vi "CreateEventGUI.vi"(8 "error in (no error)":errorcluster, 11 "DQMH_Modules":refnum<class "DQMHModuleNode.lvclass">[](array[class])) -> (0 "error out":errorcluster)   [LabVIEW 2016, in "DQMH_API.lvclass"]
uses:
  <resource>/Framework/Providers/Open_GDS/UML/DQMH_API_class/DQMH_API.lvclass
  <resource>/Framework/Providers/Open_GDS/UML/DQMHModuleNode_class/DQMHModuleNode.lvclass
  <resource>/Framework/Providers/Open_GDS/UML/DQMH_API_class/ModuleCreationType.ctl
  <resource>/Framework/Providers/Open_GDS/UML/DQMH_API_class/EventCreationType.ctl
  <resource>/Framework/Providers/Open_GDS/UML/DQMHModuleNode_class/EventType.ctl
  <vilib>/Utility/traverseref.llb/TRef TravTarget.ctl
panel:
  in  "Tree":string(tree) caption="Double click on event to create it"
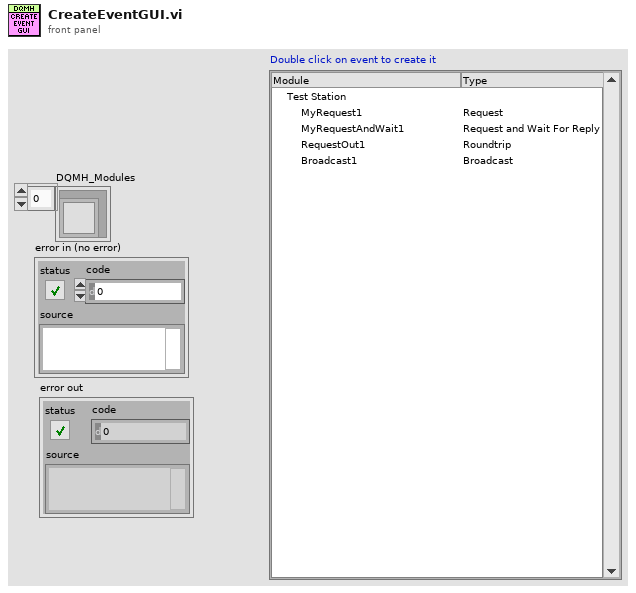
[diagram p1: front panel]
types:
  T1 = typedef "DQMH_API.lvclass/ModuleCreationType.ctl" = cluster{"LibraryName":string, "Events":T2[]}
  T2 = typedef "DQMH_API.lvclass/EventCreationType.ctl" = cluster{"Type":T3, "RequestName":string, "BroadcastName":string}
  T3 = typedef "DQMHModuleNode.lvclass/EventType.ctl" = enum16{"Request", "Request and Wait For Reply", "Roundtrip", "Broadcast"}
  T4 = cluster{"ModulesAndEvents":T1[], "EventExists":cluster{bool[]}[]}
  T5 = cluster{"Tag":string, "Cancelled":bool, "ModulesAndEvents":T1[], "ExistingEventPerModule":cluster{"Event Info":cluster{"Event VI Path":path, "Argument Path":path, "Wait Argument Path":path, "Event Arg Owner":i32, "Event Name":string, "Type":enum16{"Request", "Broadcast", "Both"}}[]}[], "EventExists":cluster{bool[]}[], "EventsCreated":cluster{bool[]}[], "DqmhCreateEventDialogRef":refnum<vi>, "Event":refnum<event-registration>, "WaitForCreation":bool, "ApplicationRef":refnum<vi>, "NewEventSubVI":refnum<vi>, "DQMH VIs":refnum<vi>[]}
  T6 = typedef "TRef TravTarget.ctl" = enum16{"FP", "BD", "Other"}
  T7 = cluster{"Event Info":cluster{"Event VI Path":path, "Argument Path":path, "Wait Argument Path":path, "Event Arg Owner":i32, "Event Name":string, "Type":enum16{"Request", "Broadcast", "Both"}}[]}[]
  T8 = cluster{"LibraryName":string, "Events":cluster{"Type":enum16{"Request", "Request and Wait For Reply", "Roundtrip", "Broadcast"}, "RequestName":string, "BroadcastName":string}[]}[]
  T9 = enum16{"Both", "Singleton Only", "Cloneable Only"}
  T10 = cluster{"Left Cell String":string, "Child Text":string[], "Child Tag":string, "Item Indent":i32, "Child Only?":bool, "Glyph Index":i32}
  T11 = enum32{"Bad", "Idle", "Run top level", "Running"}
  T12 = cluster{"Name":string, "Library":refnum<vi>, "Library Owning App":refnum<vi>, "Library Owning Folder":path, "Module Type":enum16{"Singleton", "Cloneable"}, "Public API Requests Folder":refnum<vi>, "Public API Requests Arguments Folder":refnum<vi>, "Broadcasts Folder":refnum<vi>, "Broadcasts Arguments Folder":refnum<vi>, "Obtain Broadcast Events VI":refnum<vi>, "Destroy Broadcast Events VI":refnum<vi>, "Obtain Request Events VI":refnum<vi>, "Destroy Request Events VI":refnum<vi>, "Request Events Cluster CTL":refnum<vi>, "Broadcast Events Cluster CTL":refnum<vi>, "Module Timeout VI":refnum<vi>, "Module Name VI":refnum<vi>, "Status Updated VI":refnum<vi>, "Module Not Running Error Constant VI":refnum<vi>}[]
  T13 = cluster{"Name":string, "Library":refnum<vi>, "Library Owning App":refnum<vi>, "Library Owning Folder":path, "Module Type":enum16{"Singleton", "Cloneable"}, "Public API Requests Folder":refnum<vi>, "Public API Requests Arguments Folder":refnum<vi>, "Broadcasts Folder":refnum<vi>, "Broadcasts Arguments Folder":refnum<vi>, "Obtain Broadcast Events VI":refnum<vi>, "Destroy Broadcast Events VI":refnum<vi>, "Obtain Request Events VI":refnum<vi>, "Destroy Request Events VI":refnum<vi>, "Request Events Cluster CTL":refnum<vi>, "Broadcast Events Cluster CTL":refnum<vi>, "Module Timeout VI":refnum<vi>, "Module Name VI":refnum<vi>, "Status Updated VI":refnum<vi>, "Module Not Running Error Constant VI":refnum<vi>}
  T14 = cluster{"Event VI Path":path, "Argument Path":path, "Wait Argument Path":path, "Event Arg Owner":i32, "Event Name":string, "Type":enum16{"Request", "Broadcast", "Both"}}[]
  T15 = cluster{"Event Info":cluster{"Event VI Path":path, "Argument Path":path, "Wait Argument Path":path, "Event Arg Owner":i32, "Event Name":string, "Type":enum16{"Request", "Broadcast", "Both"}}[]}
  T16 = typedef "LVRectTypeDef.ctl" = cluster{"Left":i16, "Top":i16, "Right":i16, "Bottom":i16}
  T17 = cluster{"Front Panel.Title":string, "vi reference":refnum<vi>}
  T18 = cluster{"Front Panel.Title":string, "vi reference":refnum<vi>}[]
  T19 = cluster{"value":i16, "value":i16, "value":i16, "value":i16}
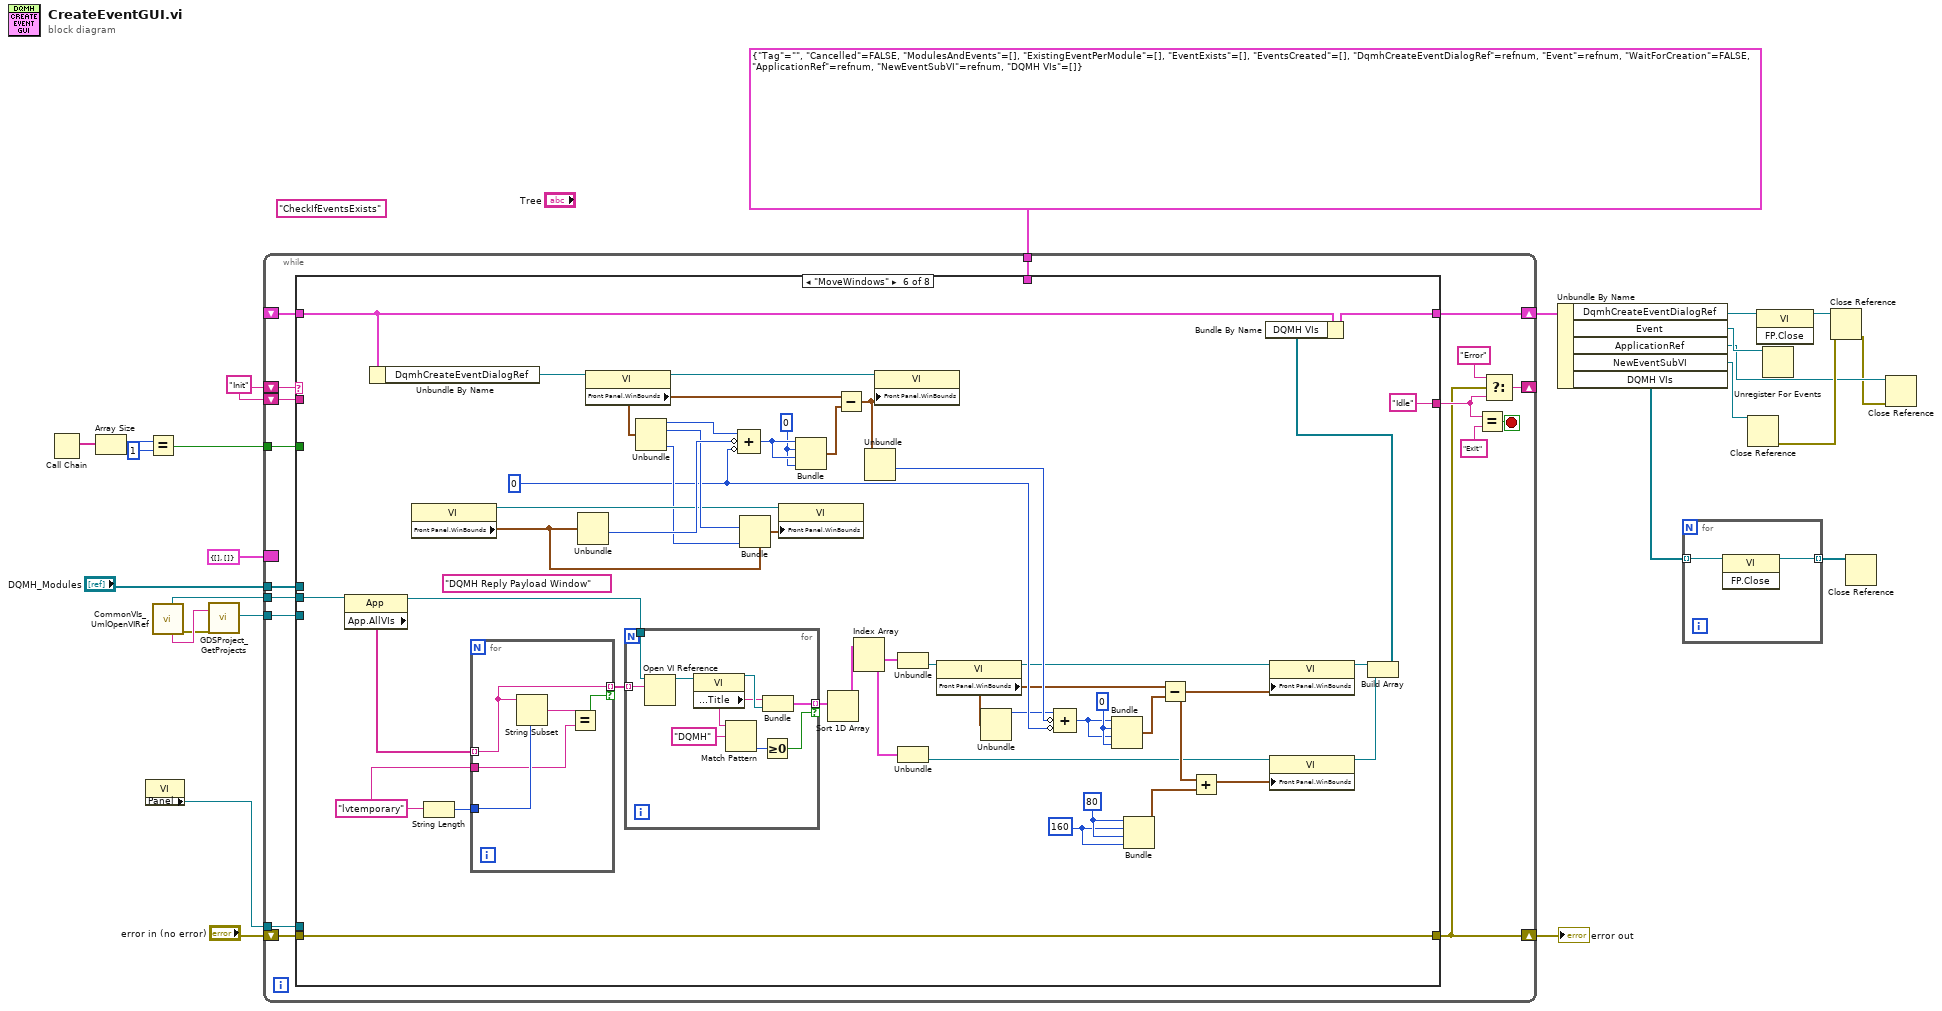
[diagram p0: block diagram]
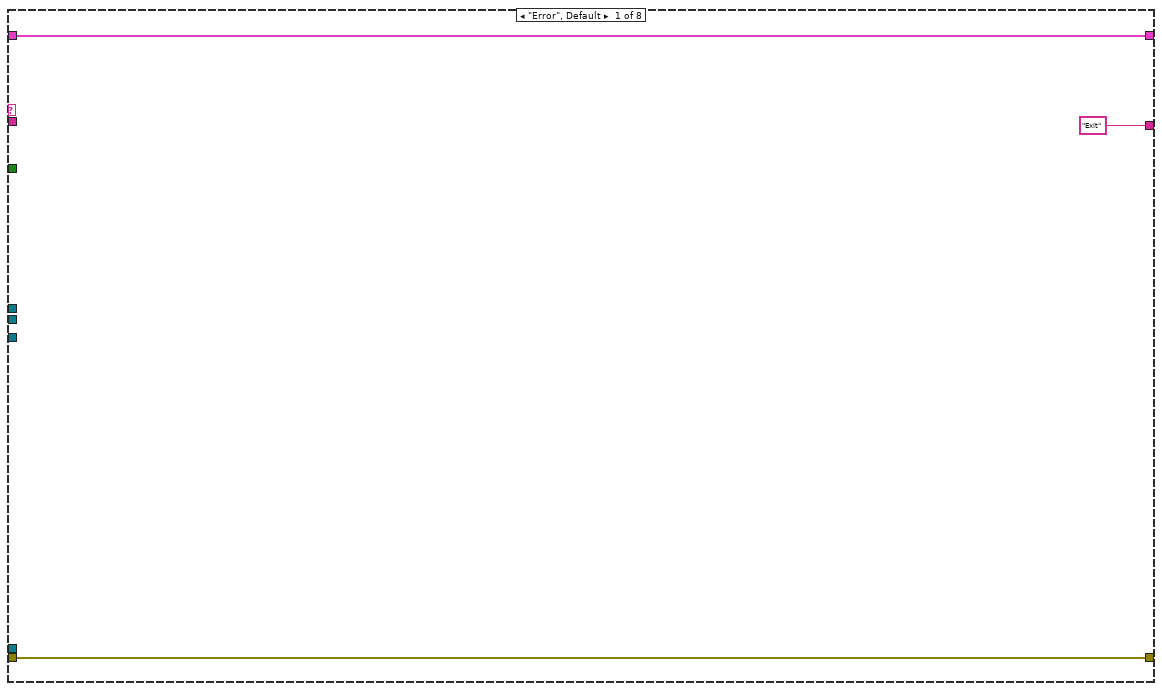
[diagram p2: hidden frame]
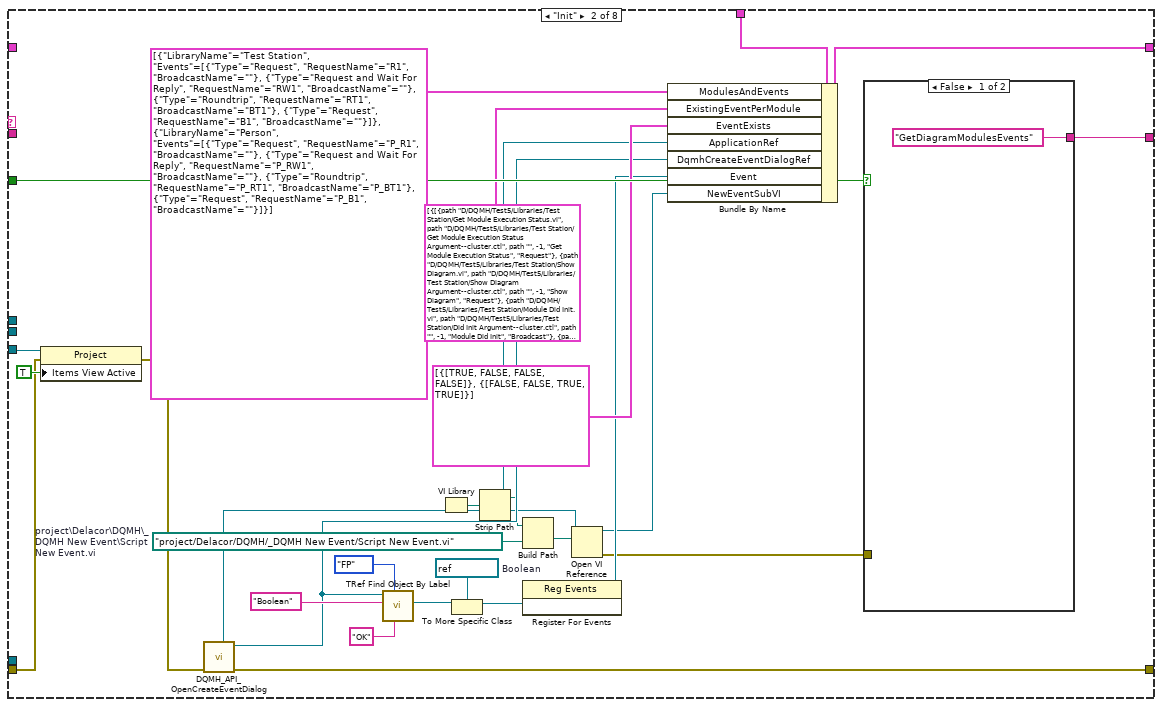
[diagram p3: hidden frame]
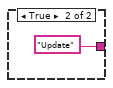
[diagram p4: hidden frame]
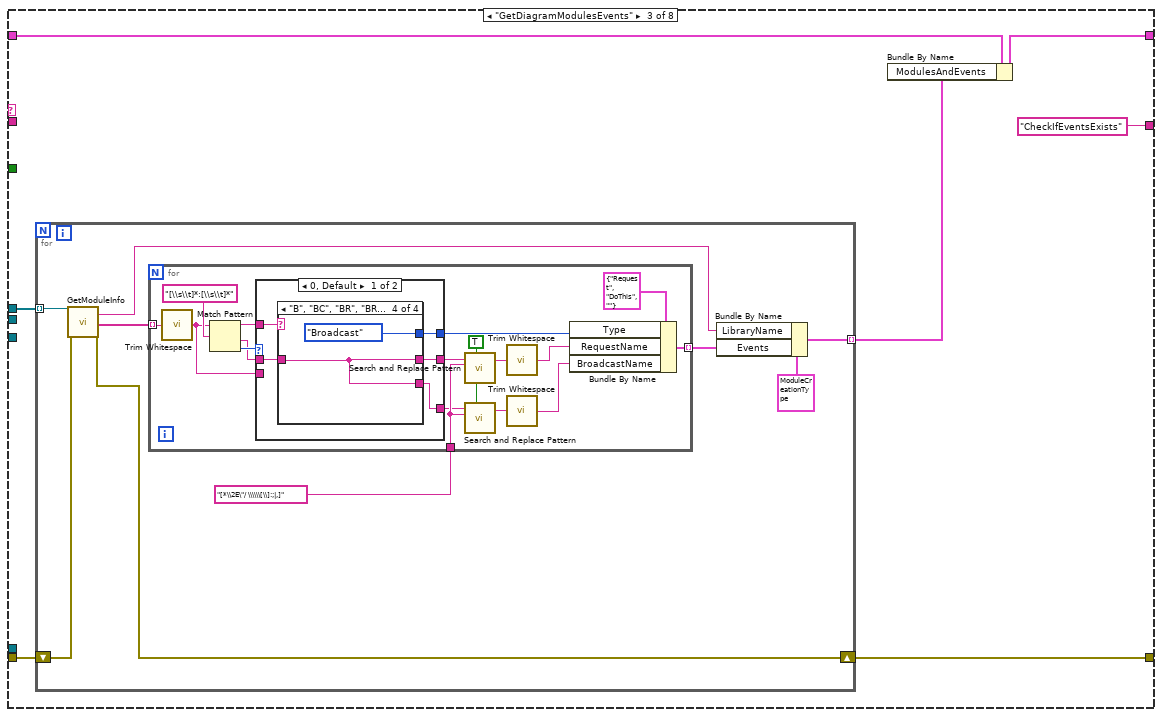
[diagram p5: hidden frame]
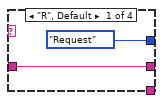
[diagram p6: hidden frame]
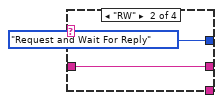
[diagram p7: hidden frame]
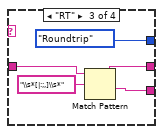
[diagram p8: hidden frame]
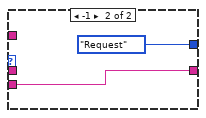
[diagram p9: hidden frame]
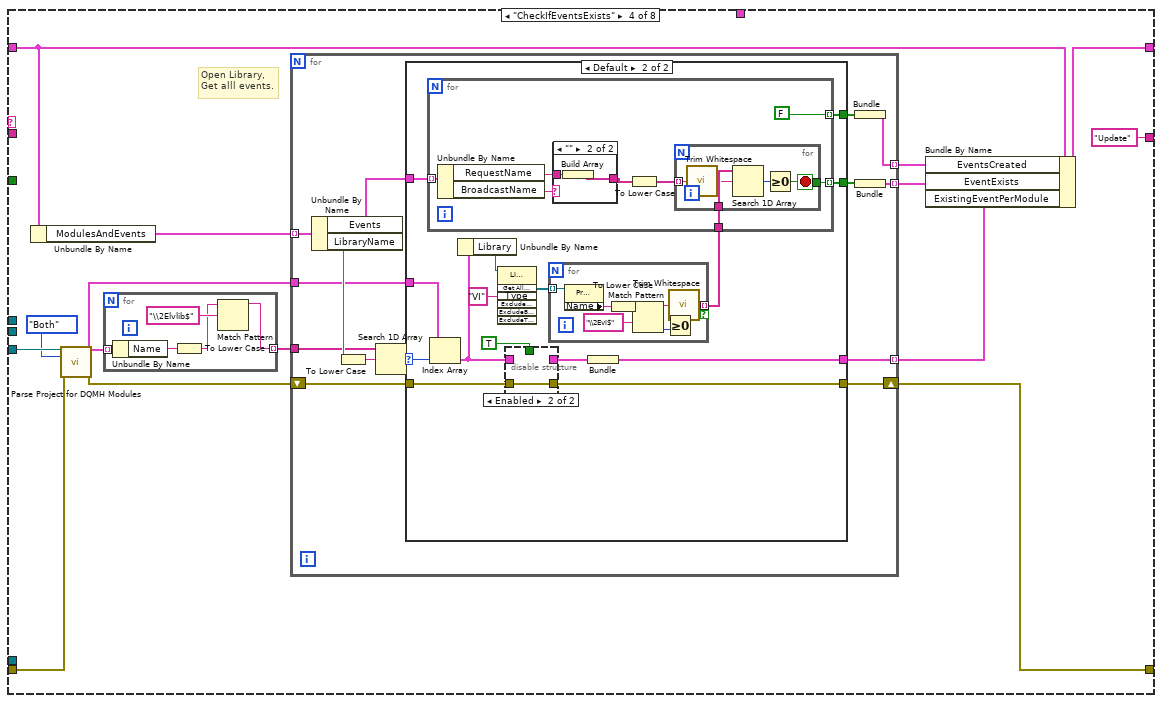
[diagram p10: hidden frame]
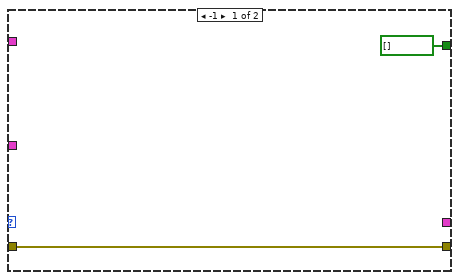
[diagram p11: hidden frame]
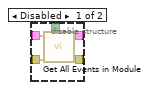
[diagram p12: hidden frame]
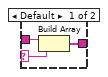
[diagram p13: hidden frame]
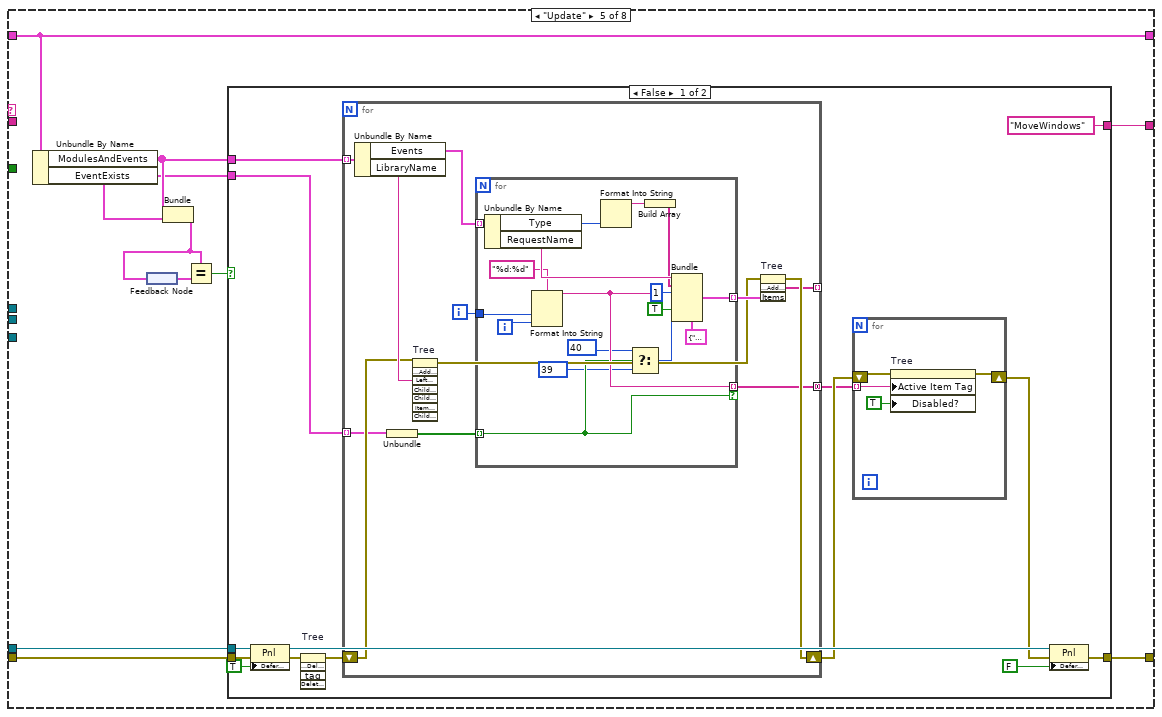
[diagram p14: hidden frame]
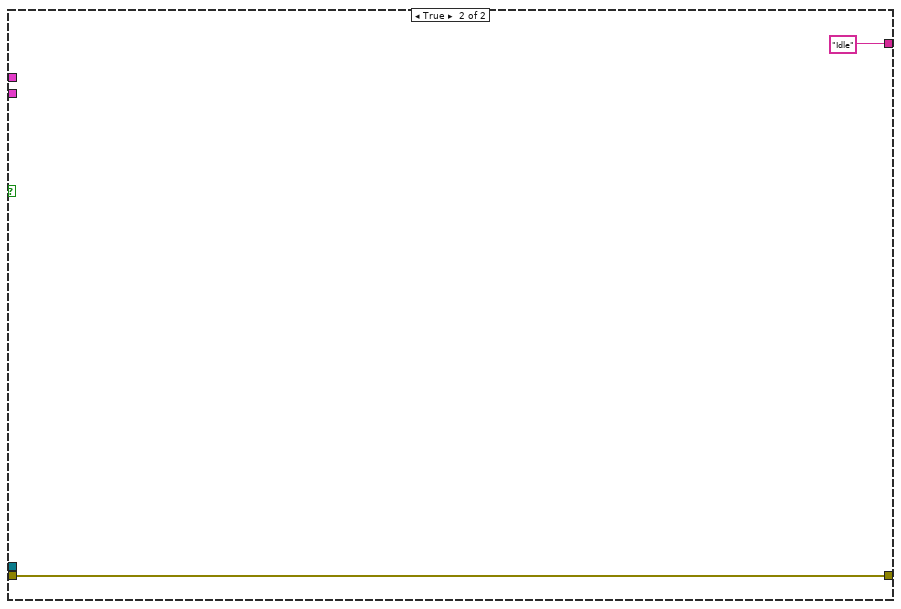
[diagram p15: hidden frame]
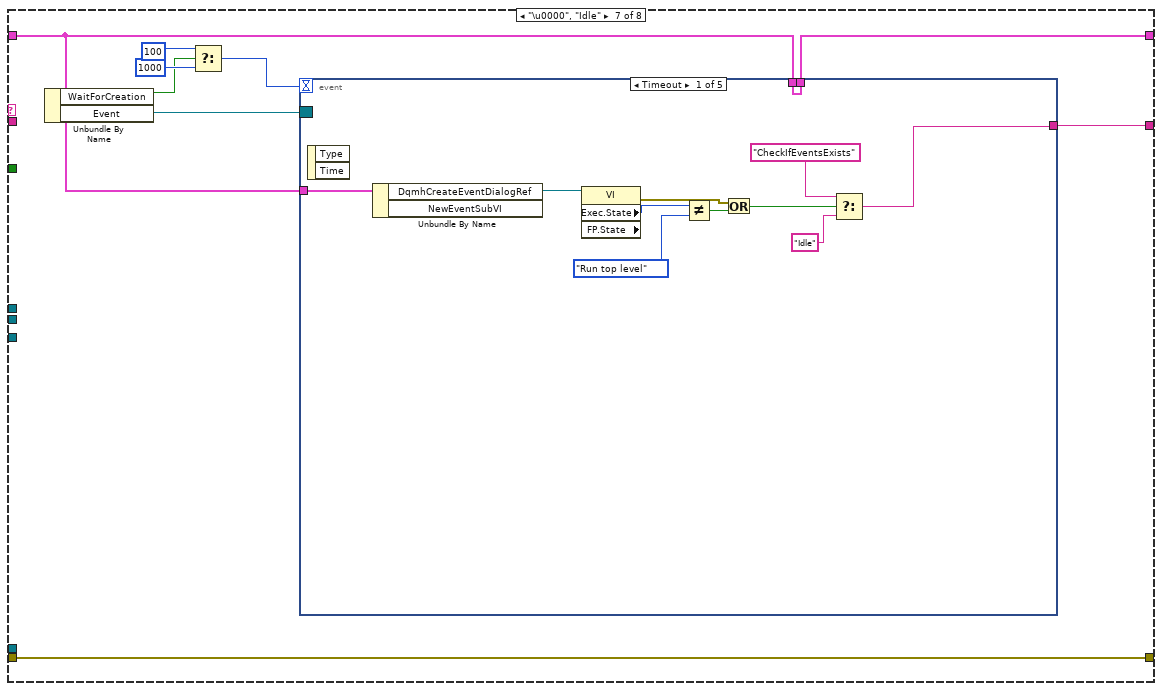
[diagram p16: hidden frame]
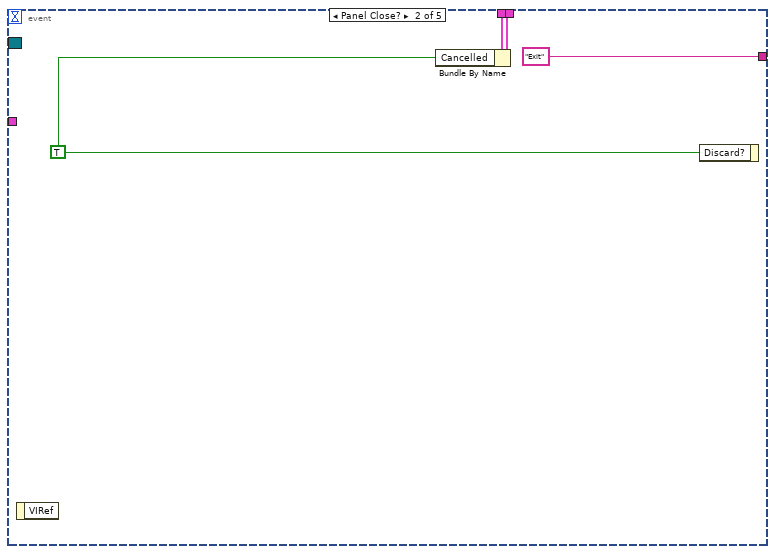
[diagram p17: hidden frame]
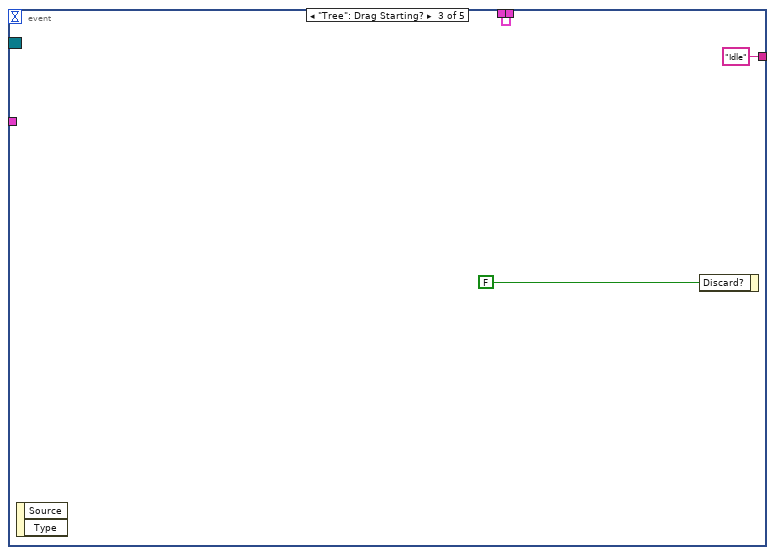
[diagram p18: hidden frame]
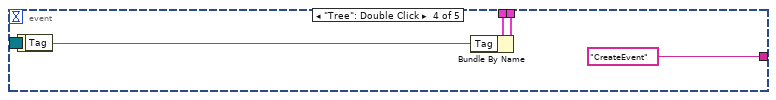
[diagram p19: hidden frame]
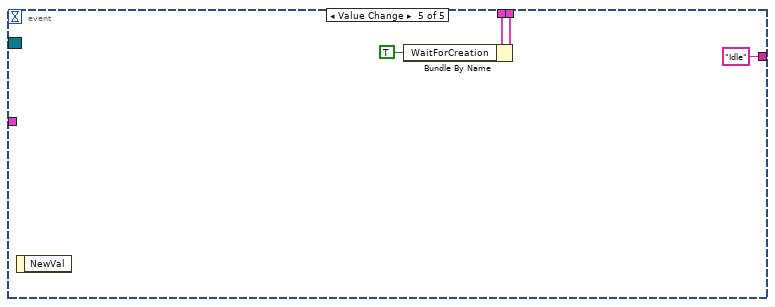
[diagram p20: hidden frame]
diagram:
  (unwired) "CheckIfEventsExists"
  w16 = "Init"
  n1 = Call Chain() -> (call chain=w15:string[])
  n2 = Array Size(array=w15) -> (size(s)=w14:i32)
  n3 = property class="VI"() -> ("Panel"=w17:refnum<vi>)  [unwired: 2 in, 2 out]
  n4 = Equal?(x=w14, y=1) -> (x = y?=w12:bool)
  n5 = call <resource>:"CommonVIs_UmlOpenVIRef.vi"() -> ("error out"=w22:errorcluster, "ProjectNameOut"=w23:string, "AppRefOut"=w7:refnum<vi>)  [unwired: 4 in, 5 out]
  n6 = call <resource>:"GDSProject_GetProjects.vi"("GetProjectRefByName"=w23, "error in (no error)"=w22) -> ("Project Refnum"=w21:refnum<vi>)  [unwired: 1 in, 16 out]
  n7 = while {
    shift-right: [w35] -> w19
    shift-left: "error in (no error)" -> [w42]
    shift-right: [w40] -> _
    shift-left: w16 -> [w41]
    shift-right: [w34] -> w25
    shift-left: _ -> [w33]
    tunnel: T5 {"Tag"="", "Cancelled"=FALSE, "ModulesAndEvents"=[], "ExistingEventPerModule"=[], "EventExists"=[], "EventsCreated"=[], "DqmhCreateEventDialogRef"=refnum, "Event"=refnum, "WaitForCreation"=FALSE, "ApplicationRef"=refnum, "NewEventSubVI"=refnum, "DQMH VIs"=[]} -> [w32]
    tunnel: w21 -> [w31]
    tunnel: "DQMH_Modules" -> [w30]
    tunnel: w17 -> [w29]
    shift-left: w16 -> [w28]
    tunnel: w12 -> [w27]
    border: T4 {"ModulesAndEvents"=[], "EventExists"=[]} -> [_]
    tunnel: w7 -> [w26]
    stop <- w39 stop-if-true
    n8 = case shown="\"MoveWindows\"" w41 {
      tunnel: w42 -> [w45 w61 w81 w129 w217 w303 w333 w364]
      tunnel: [w45 w65 w80 w128 w216 w303 w333 w368] -> w35
      tunnel: ["Exit" w72 "CheckIfEventsExists" "Update" w208 "Idle" w334 "CheckIfEventsExists"] -> w36
      tunnel: [w43 w71 w76 w131 w215 w287 w335 w369] -> w34
      tunnel: w33 -> [w43 _ w77 w138 w215 w312 w332 w366]
      tunnel: w32 -> [_ w70 _ _ _ _ _ _]
      tunnel: w31 -> [_ w64 _ w137 _ _ _ _]
      tunnel: w30 -> [_ _ w79 _ _ _ _ _]
      tunnel: w29 -> [_ _ _ _ w214 _ _ _]
      tunnel: w28 -> [_ _ _ _ _ _ _ _]
      tunnel: w27 -> [_ w69 _ _ _ _ _ _]
      tunnel: w26 -> [_ _ _ _ _ w294 _ _]
      frame "Error", Default {
      }
      frame "Init" {
        w49 = path "project/Delacor/DQMH/_DQMH New Event/Script New Event.vi"  # project\Delacor\DQMH\_DQMH New Event\Script New Event.vi
        w56 = refnum<vi> refnum  # Boolean
        n9 = property class="Project"(reference=w64, error in=w61, "Items View Active"=TRUE) -> (error out=w62:errorcluster)  [unwired: 1 out]
        n10 = call <resource>:"DQMH_API_OpenCreateEventDialog.vi"("error in (no error)"=w62) -> ("error out"=w65:errorcluster, "DqmhCreateEventDialogRef"=w54:refnum<vi>, "ApplicationRef"=w52:refnum<vi>)  [unwired: 8 in]
        n11 = call <vilib>:"TRef Find Object By Label.vi"("Label"="OK" ("Class Name"), "Traverse Target"=TRef_TravTarget."FP", "Class Name"="Boolean" ("ClassName"), "VI Ref"=w54) -> ("Found Obj Ref"=w57:refnum<vi>)  [unwired: 4 in, 3 out]
        n12 = VI Library() -> (path=w47:path)
        n13 = To More Specific Class(target class=w56, reference=w57) -> (specific class reference=w55:refnum<vi>)  [unwired: 1 in, 1 out]
        n14 = Strip Path(path=w47) -> (stripped path=w48:path)  [unwired: 1 out]
        n15 = Build Path(base path=w48, name or relative path=w49) -> (appended path=w46:path)
        n16 = register-events(w55) -> (reference out=w53:refnum<event-registration>)  [unwired: 2 in, 1 out]
        n17 = Open VI Reference(application reference (local)=w52, vi path=w46) -> (vi reference=w51:refnum<vi>, error out=w50:errorcluster)  [unwired: 4 in]
        n18 = Bundle By Name(cluster=w70, "ModulesAndEvents"=T8 [{"LibraryName"="Test Station", "Events"=[{"Type"=enum."Request", "RequestName"="R1", "BroadcastName"=""}, {"Type"=enum."Request and Wait For Reply", "RequestName"="RW1", "BroadcastName"=""}, {"Type"=enum."Roundtrip", "RequestName"="RT1", "BroadcastName"="BT1"}, {"Type"=enum."Request", "RequestName"="B1", "BroadcastName"=""}]}, {"LibraryName"="Person", "Events"=[{"Type"=enum."Request", "RequestName"="P_R1", "BroadcastName"=""}, {"Type"=enum."Request and Wait For Reply", "RequestName"="P_RW1", "BroadcastName"=""}, {"Type"=enum."Roundtrip", "RequestName"="P_RT1", "BroadcastName"="P_BT1"}, {"Type"=enum."Request", "RequestName"="P_B1", "BroadcastName"=""}]}] ("Module"), "ExistingEventPerModule"=T7 [{"Event Info"=[{"Event VI Path"=path "D:/DQMH/Test5/Libraries/Test Station/Get Module Execution Status.vi", "Argument Path"=path "D:/DQMH/Test5/Libraries/Test Station/Get Module Execution Status Argument--cluster.ctl", "Wait Argument Path"=path "", "Event Arg Owner"=-1, "Event Name"="Get Module Execution Status", "Type"=enum."Request"}, {"Event VI Path"=path "D:/DQMH/Test5/Libraries/Test Station/Show Diagram.vi", "Argument Path"=path "D:/DQMH/Test5/Libraries/Test Station/Show Diagram Argument--cluster.ctl", "Wait Argument Path"=path "", "Event Arg Owner"=-1, "Event Name"="Show Diagram", "Type"=enum."Request"}, {"Event VI Path"=path "D:/DQMH/Test5/Libraries/Test Station/Module Did Init.vi", "Argument Path"=path "D:/DQMH/Test5/Libraries/Test Station/Did Init Argument--cluster.ctl", "Wait Argument Path"=path "", "Event Arg Owner"=-1, "Event Name"="Module Did Init", "Type"=enum."Broadcast"}, {"Event VI Path"=path "D:/DQMH/Test5/Libraries/Test Station/Status Updated.vi", "Argument Path"=path "D:/DQMH/Test5/Libraries/Test Station/Status Updated Argument--cluster.ctl", "Wait Argument Path"=path "", "Event Arg Owner"=-1, "Event Name"="Status Updated", "Type"=enum."Broadcast"}, {"Event VI Path"=path "D:/DQMH/Test5/Libraries/Test Station/Error Reported.vi", "Argument Path"=path "D:/DQMH/Test5/Libraries/Test Station/Error Reported Argument--cluster.ctl", "Wait Argument Path"=path "", "Event Arg Owner"=-1, "Event Name"="Error Reported", "Type"=enum."Broadcast"}, {"Event VI Path"=path "D:/DQMH/Test5/Libraries/Test Station/Module Did Stop.vi", "Argument Path"=path "D:/DQMH/Test5/Libraries/Test Station/Stop Argument--cluster.ctl", "Wait Argument Path"=path "", "Event Arg Owner"=-1, "Event Name"="Module Did Stop", "Type"=enum."Broadcast"}, {"Event VI Path"=path "D:/DQMH/Test5/Libraries/Test Station/Update Module Execution Status.vi", "Argument Path"=path "D:/DQMH/Test5/Libraries/Test Station/Get Module Execution Status Argument--cluster.ctl", "Wait Argument Path"=path "", "Event Arg Owner"=0, "Event Name"="Update Module Execution Status", "Type"=enum."Broadcast"}]}], "EventExists"=cluster{bool[]}[] [{[TRUE, FALSE, FALSE, FALSE]}, {[FALSE, FALSE, TRUE, TRUE]}], "ApplicationRef"=w52, "DqmhCreateEventDialogRef"=w54, "Event"=w53, "NewEventSubVI"=w51) -> (w71:T5)
        n19 = case shown="False" w69 {
          tunnel: ["GetDiagramModulesEvents" "Update"] -> w72
          tunnel: w50 -> [_ _]
          frame False {
          }
          frame True {
          }
        }
      }
      frame "GetDiagramModulesEvents" {
        n20 = for {
          tunnel: w79 -> [w88] mode=indexing
          shift-right: [w85] -> w80
          shift-left: w81 -> [w89]
          tunnel: [w86] -> w75 mode=indexing
          n21 = call-dynamic "GetModuleInfo.vi"("reference in"=w88, "error in (no error)"=w89) -> ("ModuleName"=w87:string, "Events"=w90:string[], "error out"=w85:errorcluster)  [unwired: 6 in, 9 out]
          n22 = for {
            tunnel: w90 -> [w107] mode=indexing
            tunnel: "[*\\2E\"/ \\\\\\[\\]:;|,]" ("regular expression") -> [w94]
            tunnel: [w97] -> w82 mode=indexing
            w95 = TRUE ("replace all? (F)")
            n23 = call <vilib>:"Trim Whitespace.vi"("string"=w107) -> ("trimmed string"=w102:string)  [unwired: 1 in]
            n24 = Match Pattern(string=w102, regular expression="[\\s\\t]*:[\\s\\t]*") -> (before substring=w104:string, after substring=w103:string, offset past match=w105:i32)  [unwired: 1 in, 1 out]
            n25 = case shown="0, Default" w105 {
              tunnel: w103 -> [w110 _]
              tunnel: [w109 w125] -> w101
              tunnel: [w111 EventType."Request" ("Type")] -> w99
              tunnel: w104 -> [w112 _]
              tunnel: w102 -> [_ w125]
              tunnel: [w108 _] -> w93
              frame 0, Default {
                n26 = case shown="\"B\", \"BC\", \"BR\", \"BRC\"" w112 {
                  tunnel: [EventType."Request" ("Type") EventType."Request and Wait For Reply" ("Type") EventType."Roundtrip" ("Type") EventType."Broadcast" ("Type")] -> w111
                  tunnel: w110 -> [w113 w115 w119 w122]
                  tunnel: [w113 w115 w118 w122] -> w109
                  tunnel: [_ _ w117 w122] -> w108
                  frame "R", Default {
                  }
                  frame "RW" {
                  }
                  frame "RT" {
                    n27 = Match Pattern(string=w119, regular expression="\\s*[|:;,]\\s*") -> (before substring=w118:string, after substring=w117:string)  [unwired: 1 in, 2 out]
                  }
                  frame "B", "BC", "BR", "BRC" {
                  }
                }
              }
              frame -1 {
              }
            }
            n28 = call <vilib>:"Search and Replace Pattern.vi"("string"=w101, "regular expression (\"\")"=w94, "replace all? (F)"=w95) -> ("result string"=w100:string)  [unwired: 2 in, 1 out]
            n29 = call <vilib>:"Search and Replace Pattern.vi"("string"=w93, "regular expression (\"\")"=w94, "replace all? (F)"=w95) -> ("result string"=w92:string)  [unwired: 2 in, 1 out]
            n30 = call <vilib>:"Trim Whitespace.vi"("string"=w100) -> ("trimmed string"=w96:string)  [unwired: 1 in]
            n31 = call <vilib>:"Trim Whitespace.vi"("string"=w92) -> ("trimmed string"=w91:string)  [unwired: 1 in]
            n32 = Bundle By Name(cluster=T2 {"Type"=enum."Request", "RequestName"="DoThis", "BroadcastName"=""} ("Event"), "Type"=w99, "RequestName"=w96, "BroadcastName"=w91) -> (w97:T2)
          }
          n33 = Bundle By Name(cluster=T1 {"LibraryName"="TestStation", "Events"=[{"Type"=enum."Request", "RequestName"="DoThis", "BroadcastName"=""}, {"Type"=enum."Broadcast", "RequestName"="DoneIt", "BroadcastName"=""}, {"Type"=enum."Roundtrip", "RequestName"="Do", "BroadcastName"="Done"}]} ("Module"), "LibraryName"=w87, "Events"=w82) -> (w86:T1)
        }
        n34 = Bundle By Name(cluster=w77, "ModulesAndEvents"=w75) -> (w76:T5)
      }
      frame "CheckIfEventsExists" {
        # "Open Library,\nGet alll events."
        n35 = Unbundle By Name(w138) -> ("ModulesAndEvents"=w135:T1[])
        n36 = call <resource>:"Parse Project for DQMH Modules.vi"("Project (unwired: Active Project)"=w137, "Allowable Module Type"=T9."Both", "error in (no error)"=w129) -> ("DQMH Modules"=w133:T12, "error out"=w132:errorcluster)  [unwired: 6 in, 5 out]
        n37 = for {
          tunnel: w133 -> [w207] mode=indexing
          tunnel: [w203] -> w134 mode=indexing
          n38 = Unbundle By Name(w207) -> ("Name"=w206:string)
          n39 = To Lower Case(string=w206) -> (all lower case string=w204:string)
          n40 = Match Pattern(string=w204, regular expression="\\2Elvlib$") -> (before substring=w203:string)  [unwired: 1 in, 3 out]
        }
        n41 = for {
          tunnel: w135 -> [w153] mode=indexing
          tunnel: w134 -> [w151]
          tunnel: w133 -> [w149]
          tunnel: [w145] -> w130 mode=indexing
          shift-right: [w146] -> w128
          shift-left: w132 -> [w147]
          tunnel: [w142] -> w127 mode=indexing
          tunnel: [w140] -> w126 mode=indexing
          n42 = Unbundle By Name(w153) -> ("Events"=w144:T2[], "LibraryName"=w152:string)
          n43 = To Lower Case(string=w152) -> (all lower case string=w150:string)
          n44 = Search 1D Array(1D array=w151, element=w150) -> (index of element=w148:i32)  [unwired: 1 in]
          n45 = case shown="Default" w148 {
            selector: w148 -> [_ w169]
            tunnel: w149 -> [_ w170]
            tunnel: w147 -> [w155 w168]
            tunnel: [w155 w167] -> w146
            tunnel: [_ w165] -> w145
            tunnel: w144 -> [_ w159]
            tunnel: [bool[] [] w157] -> w143
            tunnel: [_ w156] -> w141
            frame -1 {
            }
            frame Default {
              n46 = Index Array(array=w170, index=w169) -> (element=w163:T13)
              n47 = Unbundle By Name(w163) -> ("Library"=w162:refnum<vi>)
              n48 = invoke class="Library" method="Get All Descendents"(reference=w162, "Type"="VI") -> ("All Descendents"=w160:refnum<vi>[])  [unwired: 5 in, 6 out]
              n49 = disable-structure shown="Enabled" {
                disable-tunnel: w168 -> [w175 w176]
                disable-tunnel: [w174 w176] -> w167
                disable-tunnel: [w173 _] -> w166
                disable-tunnel: TRUE ("include all events (F)") -> [w172 _]
                disable-tunnel: w163 -> [w171 _]
                frame Disabled {
                  n50 = call <resource>:"Get All Events in Module.vi"("include all events (F)"=w172, "error in (no error)"=w175, "Module Info"=w171) -> ("error out"=w174:errorcluster, "Event Info"=w173:T14)  [unwired: 7 in]
                }
                frame Enabled {
                }
              }
              n51 = for {
                tunnel: w160 -> [w202] mode=indexing
                tunnel: [w195] -> w158 mode=indexing if=w196
                n52 = property class="ProjectItem"(reference=w202) -> ("Name"=w201:string)  [unwired: 1 in, 2 out]
                n53 = To Lower Case(string=w201) -> (all lower case string=w200:string)
                n54 = Match Pattern(string=w200, regular expression="\\2Evi$") -> (before substring=w198:string, offset past match=w197:i32)  [unwired: 1 in, 2 out]
                n55 = Greater Or Equal To 0?(x=w197) -> (x >= 0?=w196:bool)
                n56 = call <vilib>:"Trim Whitespace.vi"("string"=w198) -> ("trimmed string"=w195:string)  [unwired: 1 in]
              }
              n57 = for {
                tunnel: w159 -> [w184] mode=indexing
                tunnel: w158 -> [w181]
                tunnel: [w179] -> w157 mode=indexing
                tunnel: [FALSE ("include all events (F)")] -> w156 mode=indexing
                n58 = Unbundle By Name(w184) -> ("RequestName"=w183:string, "BroadcastName"=w182:string)
                n59 = case shown="\"\"" w182 {
                  selector: w182 -> [w191 _]
                  tunnel: w183 -> [w192 w194]
                  tunnel: [w190 w193] -> w180
                  frame Default {
                    n60 = Build Array(w192, w191) -> (w190:string[])
                  }
                  frame "" {
                    n61 = Build Array(w194) -> (w193:string[])
                  }
                }
                n62 = To Lower Case(string=w180) -> (all lower case string=w177:string[])
                n63 = for {
                  tunnel: w181 -> [w189]
                  tunnel: w177 -> [w188] mode=indexing
                  tunnel: [w186] -> w179
                  stop <- w186 stop-if-true
                  n64 = call <vilib>:"Trim Whitespace.vi"("string"=w188) -> ("trimmed string"=w185:string)  [unwired: 1 in]
                  n65 = Search 1D Array(1D array=w189, element=w185) -> (index of element=w187:i32)  [unwired: 1 in]
                  n66 = Greater Or Equal To 0?(x=w187) -> (x >= 0?=w186:bool)
                }
              }
              n67 = Bundle("Event Info"=w166) -> (w165:T15)  [unwired: 1 in]
            }
          }
          n68 = Bundle(w141) -> (w140:cluster{bool[]})  [unwired: 1 in]
          n69 = Bundle(w143) -> (w142:cluster{bool[]})  [unwired: 1 in]
        }
        n70 = Bundle By Name(cluster=w138, "EventsCreated"=w126, "EventExists"=w127, "ExistingEventPerModule"=w130) -> (w131:T5)
      }
      frame "Update" {
        n71 = Unbundle By Name(w215) -> ("ModulesAndEvents"=w213:T1[], "EventExists"=w212:cluster{bool[]}[])
        n72 = feedback #1() -> (w211:T4)
        n73 = Bundle("ModulesAndEvents"=w213, "EventExists"=w212) -> (w210:T4)  [unwired: 1 in]
        n74 = feedback-in #1(w210) -> ()
        n75 = Equal?(x=w210, y=w211) -> (x = y?=w209:bool)
        n76 = case shown="False" w209 {
          tunnel: w217 -> [w231 w266]
          tunnel: [w228 w266] -> w216
          tunnel: w214 -> [w225 _]
          tunnel: w213 -> [w220 _]
          tunnel: w212 -> [w219 _]
          tunnel: ["MoveWindows" "Idle"] -> w208
          frame False {
            n77 = property class="Pnl"(reference=w225, error in=w231, "Defer Panel Updates"=TRUE) -> (reference out=w224:refnum<vi>, error out=w227:errorcluster)
            n78 = invoke on="Tree" class="Tree (strict)" method="Edit Tree Items.Delete"(error in=w227) -> (error out=w226:errorcluster)  [unwired: 4 in, 4 out]
            n79 = for {
              tunnel: w220 -> [w247] mode=indexing
              shift-right: [w241] -> w223
              shift-left: w226 -> [w244]
              tunnel: [w239] -> _ mode=indexing
              tunnel: [w238] -> w221 mode=concatenating
              tunnel: w219 -> [w237] mode=indexing
              i -> [w240]
              n80 = Unbundle By Name(w247) -> ("Events"=w246:T2[], "LibraryName"=w245:string)
              n81 = Unbundle(w237) -> (w236:bool[])
              n82 = invoke on="Tree" class="Tree (strict)" method="Edit Tree Items.Add Item to End"(error in=w244, "Left Cell"=w245) -> (error out=w242:errorcluster)  [unwired: 6 in, 7 out]
              n83 = for {
                tunnel: w246 -> [w264] mode=indexing
                tunnel: [w257] -> w243 mode=indexing
                tunnel: w240 -> [w249]
                tunnel: [w254] -> w238 mode=indexing if=w253
                tunnel: w236 -> [w253] mode=indexing
                i -> [w248]
                n84 = Unbundle By Name(w264) -> ("Type"=w261:T3, "RequestName"=w262:string)
                n85 = Format Into String(format string="%d:%d", w249, w248) -> (resulting string=w254:string)  [unwired: 2 in, 1 out]
                n86 = Format Into String(w261) -> (resulting string=w260:string)  [unwired: 3 in, 1 out]
                n87 = Select(t=40, s=w253, f=39) -> (s? t:f=w251:i32)
                n88 = Build Array(w260) -> (w259:string[])
                n89 = Bundle(cluster=T10 {"Left Cell String"="", "Child Text"=[], "Child Tag"="", "Item Indent"=0, "Child Only?"=FALSE, "Glyph Index"=0} ("Item"), "Left Cell String"=w262, "Child Text"=w259, "Child Tag"=w254, "Item Indent"=1, "Child Only?"=TRUE, "Glyph Index"=w251) -> (w257:T10)
              }
              n90 = invoke on="Tree" class="Tree (strict)" method="Edit Tree Items.Add Multiple Items to End"(error in=w242, "Items"=w243) -> (error out=w241:errorcluster, "Edit Tree Items:Add Multiple Items to End"=w239:string[])  [unwired: 2 in, 2 out]
            }
            n91 = for {
              shift-right: [w234] -> w222
              shift-left: w223 -> [w235]
              tunnel: w221 -> [w233] mode=indexing
              n92 = property on="Tree" class="Tree (strict)"(error in=w235, "Active Item Tag"=w233, "Disabled?"=TRUE ("Active Item:Disabled?")) -> (error out=w234:errorcluster)  [unwired: 1 in, 1 out]
            }
            n93 = property class="Pnl"(reference=w224, error in=w222, "Defer Panel Updates"=FALSE) -> (error out=w228:errorcluster)  [unwired: 1 out]
          }
          frame True {
          }
        }
      }
      frame "MoveWindows" {
        w267 = i16 160 ("value")
        w268 = i16 80 ("value")
        w284 = i16 0 ("value")
        (unwired) "DQMH Reply Payload Window" ("Front Panel.Title")
        w293 = "lvtemporary" ("regular expression")
        w305 = i16 0 ("value")
        w288 = i16 0 ("value")
        n94 = property class="App"(reference=w294) -> (reference out=w286:refnum<vi>, "App.AllVIs"=w297:string[])  [unwired: 1 in, 1 out]
        n95 = Unbundle By Name(w312) -> ("DqmhCreateEventDialogRef"=w302:refnum<vi>)
        n96 = property class="VI"() -> (reference out=w298:refnum<vi>, "Front Panel.WinBounds"=w301:T16)  [unwired: 2 in, 1 out]
        n97 = String Length(string=w293) -> (length=w296:i32)
        n98 = for {
          tunnel: w297 -> [w323] mode=indexing
          tunnel: w296 -> [w326]
          tunnel: w293 -> [w324]
          tunnel: [w323] -> w295 mode=indexing if=w322
          n99 = String Subset(string=w323, length (rest)=w326) -> (substring=w325:string)  [unwired: 1 in]
          n100 = Equal?(x=w325, y=w324) -> (x = y?=w322:bool)
        }
        n101 = Unbundle(w301) -> ("Right"=w309:i16)  [unwired: 3 out]
        n102 = property class="VI"(reference=w302) -> (reference out=w307:refnum<vi>, "Front Panel.WinBounds"=w308:T16)  [unwired: 1 in, 1 out]
        n103 = for {
          tunnel: w295 -> [w321] mode=indexing
          tunnel: [w318] -> w292 mode=indexing if=w313
          tunnel: w286 -> [w317]
          n104 = Open VI Reference(application reference (local)=w317, vi path=w321) -> (vi reference=w320:refnum<vi>)  [unwired: 4 in, 1 out]
          n105 = property class="VI"(reference=w320) -> (reference out=w319:refnum<vi>, "Front Panel.Title"=w316:string)  [unwired: 1 in, 1 out]
          n106 = Match Pattern(string=w316, regular expression="DQMH") -> (offset past match=w314:i32)  [unwired: 1 in, 3 out]
          n107 = Greater Or Equal To 0?(x=w314) -> (x >= 0?=w313:bool)
          n108 = Bundle("Front Panel.Title"=w316, "vi reference"=w319) -> (w318:T17)  [unwired: 1 in]
        }
        n109 = Unbundle(w308) -> ("Left"=w310:i16, "Top"=w300:i16, "Bottom"=w290:i16)  [unwired: 1 out]
        n110 = Compound Arithmetic op=ADD(w310, invert w309, invert w288) -> (w306:i16)
        n111 = Bundle(cluster=w301, "Top"=w300, "Bottom"=w290) -> (w299:T16)  [unwired: 2 in]
        n112 = property class="VI"(reference=w298, "Front Panel.WinBounds"=w299) -> ()  [unwired: 1 in, 2 out]
        n113 = Bundle(w306, "value"=w305, w306, "value"=w305) -> (w304:cluster{i16, "value":i16, i16, "value":i16})  [unwired: 1 in]
        n114 = Sort 1D Array(array=w292) -> (sorted array=w269:T18)
        n115 = Subtract(x=w308, y=w304) -> (x-y=w291:T16)
        n116 = Index Array(array=w269) -> (element #1=w277:T17, element #2=w276:T17)  [unwired: 2 in]
        n117 = Unbundle(w291) -> ("Right"=w289:i16)  [unwired: 3 out]
        n118 = property class="VI"(reference=w307, "Front Panel.WinBounds"=w291) -> ()  [unwired: 1 in, 2 out]
        n119 = Unbundle(w277) -> ("vi reference"=w279:refnum<vi>)  [unwired: 1 out]
        n120 = Unbundle(w276) -> ("vi reference"=w272:refnum<vi>)  [unwired: 1 out]
        n121 = property class="VI"(reference=w279) -> (reference out=w282:refnum<vi>, "Front Panel.WinBounds"=w281:T16)  [unwired: 1 in, 1 out]
        n122 = Unbundle(w281) -> ("Left"=w280:i16)  [unwired: 3 out]
        n123 = Compound Arithmetic op=ADD(w280, invert w289, invert w288) -> (w283:i16)
        n124 = Bundle(w283, "value"=w284, w283, "value"=w284) -> (w285:cluster{i16, "value":i16, i16, "value":i16})  [unwired: 1 in]
        n125 = Bundle("value"=w268, "value"=w267, "value"=w268, "value"=w267) -> (w278:T19)  [unwired: 1 in]
        n126 = Subtract(x=w281, y=w285) -> (x-y=w273:T16)
        n127 = Add(x=w273, y=w278) -> (x+y=w271:T16)
        n128 = property class="VI"(reference=w282, "Front Panel.WinBounds"=w273) -> (reference out=w275:refnum<vi>)  [unwired: 1 in, 1 out]
        n129 = property class="VI"(reference=w272, "Front Panel.WinBounds"=w271) -> (reference out=w270:refnum<vi>)  [unwired: 1 in, 1 out]
        n130 = Build Array(w275, w270) -> (w274:refnum<vi>[])
        n131 = Bundle By Name(cluster=w312, "DQMH VIs"=w274) -> (w287:T5)
      }
      frame "\u0000", "Idle" {
        n132 = Unbundle By Name(w332) -> ("WaitForCreation"=w327:bool, "Event"=w331:refnum<event-registration>)
        n133 = Select(t=100, s=w327, f=1000) -> (s? t:f=w328:i32)
        n134 = event shown="[0] Timeout" {
          selector: w331 -> [_ _ _ _ _]
          dyn-events: _ -> [_ _ _ _ _]
          timeout: w328 -> [_ _ _ _ _]
          tunnel: w332 -> [w346 w349 w352 w357 w361]
          tunnel: [w346 w348 w352 w355 w360] -> w335
          tunnel: [w338 "Exit" "Idle" ("f") "CreateEvent" "Idle" ("f")] -> w334
          tunnel: w332 -> [w345 _ _ _ _]
          event Timeout {
            n135 = event-data() -> ()  [unwired: 1 in, 2 out]
            n136 = Unbundle By Name(w345) -> ("DqmhCreateEventDialogRef"=w336:refnum<vi>)  [unwired: 1 out]
            n137 = property class="VI" props=["Exec.State", "FP.State"](reference=w336) -> (error out=w342:errorcluster, "Exec.State"=w337:T11)  [unwired: 1 in, 2 out]
            n138 = Not Equal?(x=w337, y=T11."Run top level") -> (x != y?=w343:bool)
            n139 = Or(x=w342, y=w343) -> (x .or. y?=w341:bool)
            n140 = Select(t="CheckIfEventsExists", s=w341, f="Idle") -> (s? t:f=w338:string)
          }
          event Panel Close? {
            w347 = TRUE ("Discard?")
            n141 = event-data() -> ()  [unwired: 1 in, 1 out]
            n142 = Bundle By Name(cluster=w349, "Cancelled"=w347) -> (w348:T5)
            n143 = event-data("Discard?"=w347) -> ()  [unwired: 1 in, 1 out]
          }
          event "Tree": Drag Starting? {
            n144 = event-data() -> ()  [unwired: 1 in, 2 out]
            n145 = event-data("Discard?"=FALSE) -> ()  [unwired: 1 in, 1 out]
          }
          event "Tree": Double Click {
            n146 = event-data() -> ("Tag"=w354:string)  [unwired: 1 in]
            n147 = Bundle By Name(cluster=w357, "Tag"=w354) -> (w355:T5)
          }
          event Value Change {
            n148 = event-data() -> ()  [unwired: 1 in, 1 out]
            n149 = Bundle By Name(cluster=w361, "WaitForCreation"=TRUE) -> (w360:T5)
          }
        }
      }
      frame "CreateEvent" {
        n150 = Unbundle By Name(w366) -> ("Tag"=w374:string)
        n151 = Unbundle By Name(w366) -> ("DqmhCreateEventDialogRef"=w365:refnum<vi>)
        n152 = Unbundle By Name(w366) -> ("EventsCreated"=w373:cluster{bool[]}[], "ModulesAndEvents"=w379:T1[])
        n153 = Scan From String(format string="%d:%d", input string=w374) -> (output 1=w371:i32, output 2=w370:i32)  [unwired: 4 in, 3 out]
        n154 = Index Array(array=w379, index=w371) -> (element=w378:T1)
        n155 = Unbundle By Name(w378) -> ("LibraryName"=w376:string, "Events"=w377:T2[])
        n156 = in-place {
          in-place-border: w370 -> [w404]
          n157 = in-place-array #2(w373, w371) -> (w406:cluster{bool[]})
          n158 = Unbundle(w406) -> (w405:bool[])
          n159 = Replace Array Subset(array=w405, new element=TRUE ("new element/subarray"), index=w404) -> (w402:bool[])
          n160 = Bundle(w402) -> (w401:cluster{bool[]})  [unwired: 1 in]
          n161 = in-place-array #2(w401) -> ()  [unwired: 2 out]
        }
        n162 = Index Array(array=w377, index=w370) -> (element=w375:T2)
        n163 = disable-structure shown="Enabled" {
          disable-tunnel: w364 -> [w399 w400]
          disable-tunnel: [w398 w400] -> w363
          frame Disabled {
            n164 = call <vilib>:"Set Busy.vi"("error in (no error)"=w399) -> ("error out"=w398:errorcluster)  [unwired: 9 in, 1 out]
          }
          frame Enabled {
          }
        }
        n165 = call <resource>:"DQMH_API_RunCreateEventDialog.vi"("error in (no error)"=w363, "Event"=w375, "ModuleName"=w376) -> ("error out"=w367:errorcluster, "ViRef"=w362:refnum<vi>)  [unwired: 7 in]
        n166 = disable-structure shown="Enabled" {
          disable-tunnel: [w387 w394] -> w369
          disable-tunnel: [w385 w396] -> w368
          disable-tunnel: w367 -> [w384 w396]
          disable-tunnel: w366 -> [w383 w395]
          disable-tunnel: w365 -> [w382 w393]
          disable-tunnel: w362 -> [_ w391]
          frame Disabled {
            n167 = Close Reference(reference=w382, error in (no error)=w384) -> (error out=w381:errorcluster)
            n168 = flat-sequence {
              tunnel: [w390] -> w386
              tunnel: [w389] -> w385
              tunnel: w384 -> [w388]
              tunnel: w381 -> [_]
              frame #0 {
                n169 = call <vilib>:"Unset Busy.vi"() -> ()  [unwired: 11 in, 1 out]
                n170 = call <resource>:"DQMH_API_OpenCreateEventDialog.vi"("error in (no error)"=w388) -> ("error out"=w389:errorcluster, "DqmhCreateEventDialogRef"=w390:refnum<vi>)  [unwired: 8 in, 1 out]
              }
            }
            n171 = Bundle By Name(cluster=w383, "DqmhCreateEventDialogRef"=w386) -> (w387:T5)
          }
          frame Enabled {
            n172 = Not Equal?(x=w391, y=w393) -> (x != y?=w392:bool)
            n173 = case shown="True" w392 {
              tunnel: w391 -> [_ w397]
              frame False {
              }
              frame True {
                n174 = Close Reference(reference=w397) -> ()  [unwired: 1 in, 1 out]
              }
            }
            n175 = Bundle By Name(cluster=w395, "DqmhCreateEventDialogRef"=w391) -> (w394:T5)
          }
        }
      }
    }
    n176 = Equal?(x=w36, y="Exit") -> (x = y?=w39:bool)
    n177 = Select(t="Error", s=w35, f=w36) -> (s? t:f=w40:string)
  }
  "error out" <- w19
  n178 = Unbundle By Name(w25) -> ("DqmhCreateEventDialogRef"=w11:refnum<vi>, "Event"=w8:refnum<event-registration>, "ApplicationRef"=w4:refnum<vi>, "NewEventSubVI"=w6:refnum<vi>, "DQMH VIs"=w2:refnum<vi>[])
  n179 = for {
    tunnel: w2 -> [w408] mode=indexing
    tunnel: [w407] -> w1 mode=indexing
    n180 = invoke class="VI" method="FP.Close"(reference=w408) -> (reference out=w407:refnum<vi>)  [unwired: 2 in, 2 out]
  }
  n181 = Close Reference(reference=w6) -> (error out=w5:errorcluster)  [unwired: 1 in]
  n182 = invoke class="VI" method="FP.Close"(reference=w11) -> (reference out=w10:refnum<vi>)  [unwired: 2 in, 2 out]
  n183 = Unregister For Events(event registration refnum=w8) -> ()  [unwired: 1 in, 1 out]
  n184 = Close Reference(reference=w10, error in (no error)=w5) -> (error out=w3:errorcluster)
  n185 = Close Reference(reference=w1) -> ()  [unwired: 1 in, 1 out]
  n186 = Close Reference(reference=w4, error in (no error)=w3) -> ()  [unwired: 1 out]
